vi "client_tcp.vi"() -> ()   [LabVIEW 2016]
panel:
  in  "Clear":bool
  out "wynik dzialania 2":cluster{"Y":dbl[], "Y":dbl[]}[](graph)
  in  "Stop":bool
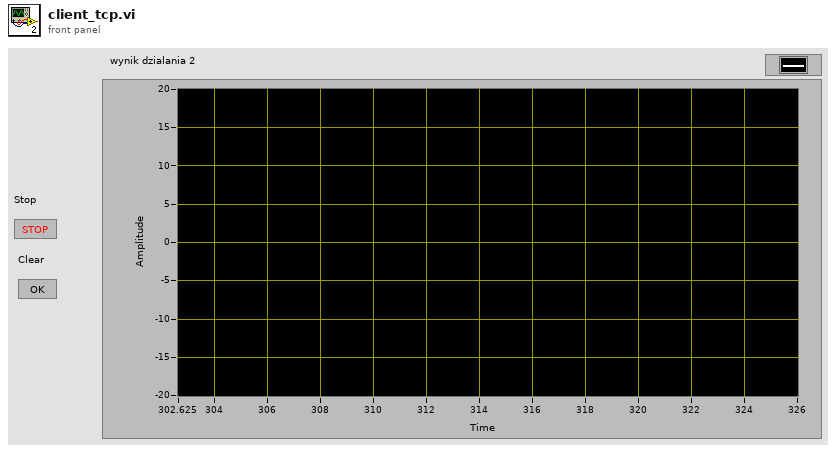
[diagram p1: front panel]
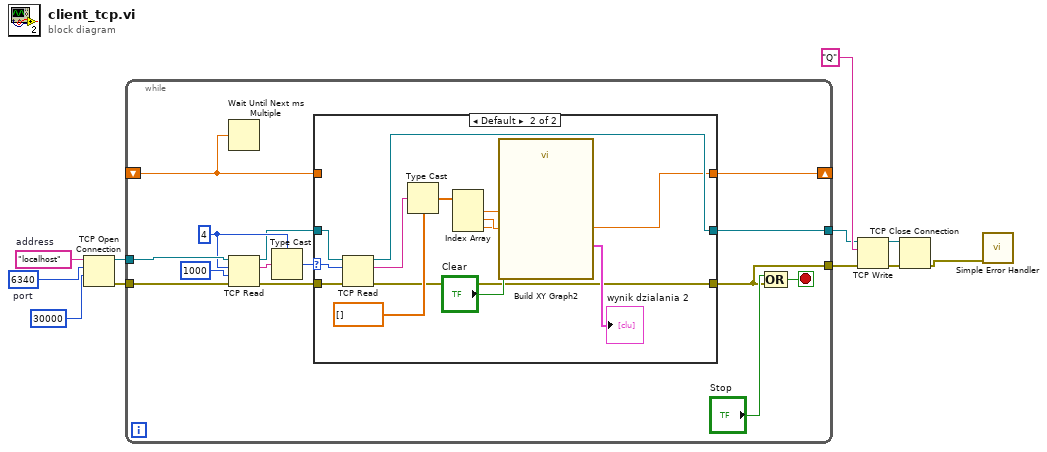
[diagram p0: block diagram]
diagram:
  w10 = u16 6340  # port
  w11 = "localhost"  # address
  n1 = TCP Open Connection(address=w11, remote port or service name=w10, timeout ms (60000)=30000) -> (connection ID=w8:refnum<k5>, error out=w9:errorcluster)  [unwired: 2 in]
  n2 = while {
    tunnel: w9 -> [w20]
    tunnel: w8 -> [w21]
    tunnel: [w16] -> w4
    tunnel: [w15] -> w3
    shift-right: [w13] -> _
    shift-left: _ -> [w12]
    stop <- w24 stop-if-true
    w19 = 4
    n3 = Wait Until Next ms Multiple(millisecond multiple=w12) -> ()  [unwired: 1 out]
    n4 = TCP Read(connection ID=w21, bytes to read=w19, error in (no error)=w20, 9:1000 ("timeout ms (25000)")) -> (connection ID out=w17:refnum<k5>, data out=w22:string, error out=w18:errorcluster)  [unwired: 1 in]
    n5 = Type Cast(type=w19, x=w22) -> (*(type *) &x=w23:i32)
    n6 = case shown="Default" w23 {
      selector: w23 -> [_ w30]
      tunnel: [w28 w31] -> w15
      tunnel: w18 -> [w28 w38]
      tunnel: w17 -> [w27 w37]
      tunnel: [w27 w36] -> w16
      tunnel: [w26 w29] -> w13
      tunnel: w12 -> [w26 _]
      frame ..0 {
      }
      frame Default {
        n7 = TCP Read(connection ID=w37, bytes to read=w30, error in (no error)=w38) -> (connection ID out=w36:refnum<k5>, data out=w40:string, error out=w31:errorcluster)  [unwired: 2 in]
        n8 = Type Cast(type=dbl[] [], x=w40) -> (*(type *) &x=w41:dbl[])
        n9 = Index Array(array=w41) -> (element #1=w33:dbl, element #2=w32:dbl, element #3=w29:dbl)  [unwired: 3 in]
        n10 = call "Build XY Graph2"("Reset"="Clear", "Y Input"=w32, "X Input"=w33) -> ("XY Graph"=→"wynik dzialania 2":cluster{"Y":dbl[], "Y":dbl[]}[])  [unwired: 7 in, 1 out]
      }
    }
    n11 = Compound Arithmetic op=OR("Stop", w15) -> (w24:bool)
  }
  n12 = TCP Write(connection ID=w4, data in="Q", error in (no error)=w3) -> (connection ID out=w7:refnum<k5>, error out=w6:errorcluster)  [unwired: 2 out]
  n13 = TCP Close Connection(connection ID=w7, error in (no error)=w6) -> (error out=w2:errorcluster)  [unwired: 1 in, 1 out]
  n14 = call <vilib>:"Simple Error Handler.vi"("error in (no error)"=w2) -> ()  [unwired: 4 in, 5 out]
